vi "Create All Message Queues v00.vi"(8 "error in (no error)":T1 caption="Fehler (Eingang, kein Fehler)") -> (0 "error out":T1 caption="Fehler (Ausgang)", 3 "Nachrichten-Queues (Ausgang)":T2)   [LabVIEW 2014, in "Message Queue.lvlib"]
doc: "Dieses VI erstellt und initialisiert alle Nachrichten-Queues Ihrer Anwendung. Klicken Sie zum Hinzufügen von Nachrichten-Queues mit der rechten Maustaste auf die Konstante \"Nachrichten-Queues\" und wählen Sie \"Typdefinition öffnen\". Fügen Sie die neue(n) Queue(s) der Typdefinition hinzu und initialisieren Sie sie in diesem VI."
uses:
  Documents/LabVIEW Data/Unbenanntes Projekt 8/support/Message Queue/Message Queue.lvlib
  All Message Queues.ctl
  Documents/LabVIEW Data/Unbenanntes Projekt 8/support/Message Queue/Message Cluster.ctl
  Documents/LabVIEW Data/Unbenanntes Projekt 8/support/Message Queue/Enqueue Message (Single).vi
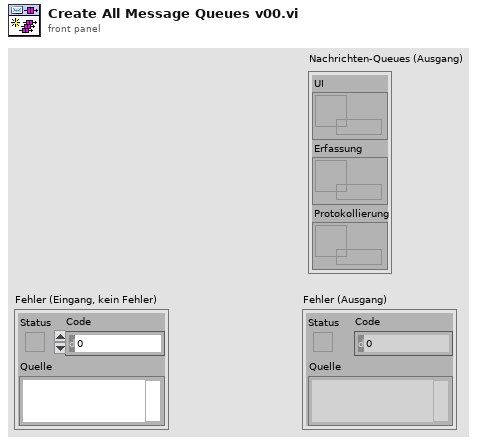
[diagram p1: front panel]
types:
  T1 = cluster{"Status":bool, "Code":i32, "Quelle":string}
  T2 = typedef "Message Queue.lvlib/All Message Queues.ctl" = cluster{"UI":refnum<queue>, "Erfassung":refnum<queue>, "Traverse":refnum<queue>}
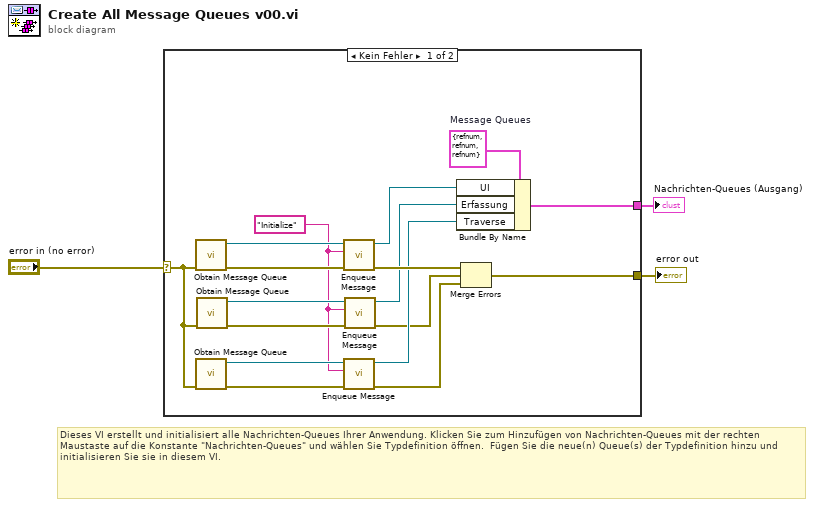
[diagram p0: block diagram]
diagram:
  # "Dieses VI erstellt und initialisiert alle Nachrichten-Queues Ihrer Anwendung. Klicken Sie zum Hinzufügen von Nachrichten-Queues mit der rechten Maustaste auf die Konstante \"Nachrichten-Queues\" und wählen Sie Typdefinition öffnen.  Fügen Sie die neue(n) Queue(s) der Typdefinition hinzu und initialisieren Sie sie in diesem VI."
  n1 = case shown="Kein Fehler" "error in (no error)" {
    selector: "error in (no error)" -> [w11 w21]
    tunnel: [w6 w21] -> w3
    tunnel: [w18 _] -> w2
    frame No Error {
      w10 = "Initialize" ("Message")
      w19 = T2 {"UI"=refnum, "Erfassung"=refnum, "Traverse"=refnum}  # Message Queues
      n2 = call "Obtain Message Queue.vi"("error in (no error)"=w11) -> ("error out"=w17:T1, "Nachrichten-Queue"=w16:refnum<queue>)  [unwired: 9 in]
      n3 = call "Obtain Message Queue.vi"("error in (no error)"=w11) -> ("error out"=w13:T1, "Nachrichten-Queue"=w12:refnum<queue>)  [unwired: 9 in]
      n4 = call "Obtain Message Queue.vi"("error in (no error)"=w11) -> ("error out"=w14:T1, "Nachrichten-Queue"=w15:refnum<queue>)  [unwired: 9 in]
      n5 = call-poly "Enqueue Message.vi"("error in (no error)"=w17, "Nachricht"=w10, "Nachrichten-Queue"=w16) -> ("error out"=w20:T1, "Nachrichten-Queue (Kopie)"=w9:refnum<queue>)  [unwired: 7 in]
      n6 = call-poly "Enqueue Message.vi"("error in (no error)"=w13, "Nachricht"=w10, "Nachrichten-Queue"=w12) -> ("error out"=w4:T1, "Nachrichten-Queue (Kopie)"=w7:refnum<queue>)  [unwired: 7 in]
      n7 = call-poly "Enqueue Message.vi"("error in (no error)"=w14, "Nachricht"=w10, "Nachrichten-Queue"=w15) -> ("error out"=w5:T1, "Nachrichten-Queue (Kopie)"=w8:refnum<queue>)  [unwired: 7 in]
      n8 = Bundle By Name(cluster=w19, "UI"=w9, "Erfassung"=w8, "Traverse"=w7) -> (w18:T2)
      n9 = Merge Errors(w20, w5, w4) -> (w6:errorcluster)
    }
    frame Error {
    }
  }
  "Nachrichten-Queues (Ausgang)" <- w2
  "error out" <- w3
